vi "Flatten User Events to Variant.vi"(8 "error in (no error)":errorcluster, 9 "All User Events":refnum<user-event>[](array[refnum]), 10 "All User Event Names":string[](array[string]), 11 "Quit Event":refnum<user-event>) -> (0 "error out":errorcluster, 3 "Variant":variant)   [LabVIEW 2011]
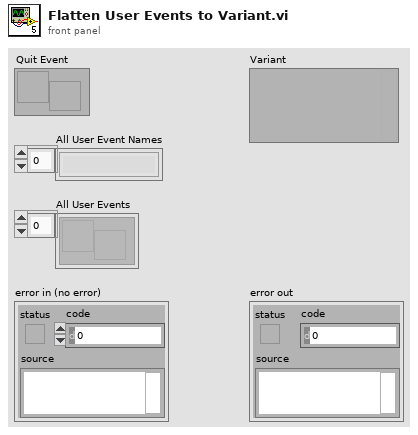
[diagram p1: front panel]
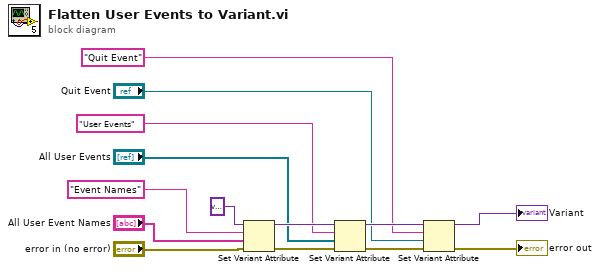
[diagram p0: block diagram]
diagram:
  n1 = Set Variant Attribute(Variant=variant ("variant"), name="Event Names" ("Tag"), value="All User Event Names", error in="error in (no error)") -> (Variant out=w11:variant, error out=w10:errorcluster)  [unwired: 1 out]
  n2 = Set Variant Attribute(Variant=w11, name="User Events" ("Tag"), value="All User Events", error in=w10) -> (Variant out=w8:variant, error out=w9:errorcluster)  [unwired: 1 out]
  n3 = Set Variant Attribute(Variant=w8, name="Quit Event" ("Tag"), value="Quit Event", error in=w9) -> (Variant out=→"Variant":variant, error out=→"error out":errorcluster)  [unwired: 1 out]
